vi "Helper SubVI - Get Peak Signal-to-noise Ratio (PNSR).vi"(10 "dest":dbl[][](array[numeric]), 11 "source":dbl[][](array[numeric])) -> (3 "PSNR (dB)":dbl)   [LabVIEW 2023]
doc: "Computes the peak signal-to-noise ratio (PNSR) of the reconstructed image."
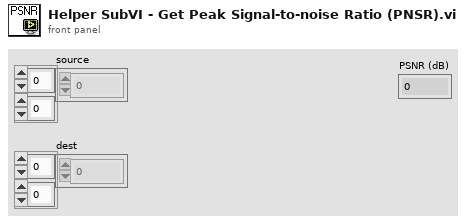
[diagram p1: front panel]
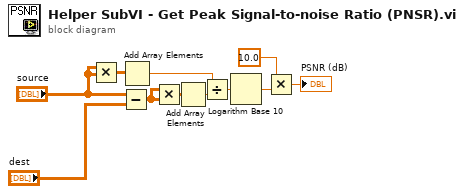
[diagram p0: block diagram]
diagram:
  n1 = Multiply(x="source", y="source") -> (x*y=w6:dbl[][])
  n2 = Subtract(x="source", y="dest") -> (x-y=w7:dbl[][])
  n3 = Add Array Elements(numeric array=w6) -> (sum=w1:dbl)
  n4 = Multiply(x=w7, y=w7) -> (x*y=w8:dbl[][])
  n5 = Add Array Elements(numeric array=w8) -> (sum=w5:dbl)
  n6 = Divide(x=w1, y=w5) -> (x/y=w4:dbl)
  n7 = Logarithm Base 10(1:w4) -> (0:w3:dbl)
  n8 = Multiply(x=10.0, y=w3) -> (x*y=→"PSNR (dB)":dbl)
